vi "Saving Ascan data.vi"(8 "error in (no error)":errorcluster caption="错误输入（无错误）", 10 "Ascan Data":dbl[](array[numeric]) caption="第一行", 11 "名称或相对路径":string) -> (0 "error out":errorcluster caption="错误输出")   [LabVIEW 2015, in "Utility VIs.lvlib"]
uses:
  Utility VIs.lvlib
  <vilib>/Utility/file.llb/Write Delimited Spreadsheet (DBL).vi
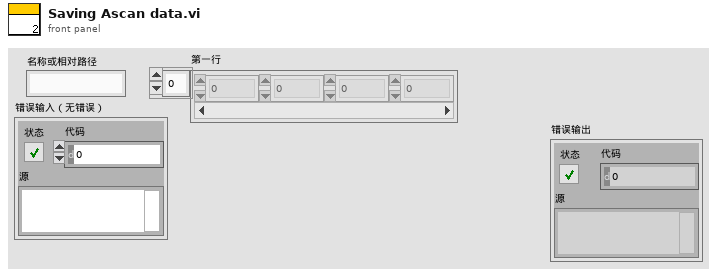
[diagram p1: front panel]
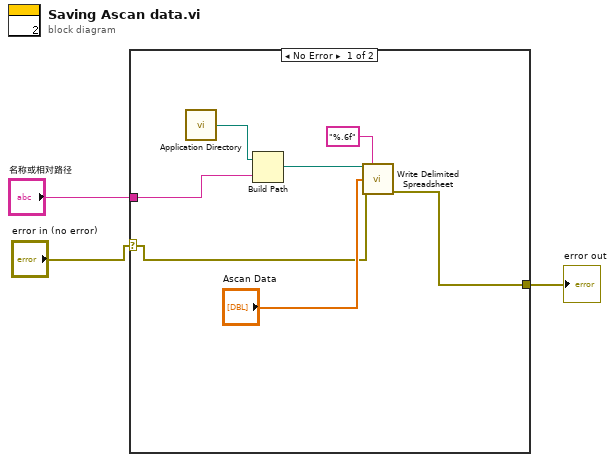
[diagram p0: block diagram]
diagram:
  n1 = case shown="No Error" "error in (no error)" {
    selector: "error in (no error)" -> [w5 w11]
    tunnel: "名称或相对路径" -> [w9 _]
    tunnel: [w7 w11] -> w2
    frame No Error {
      n2 = call <vilib>:"Application Directory.vi"() -> ("Application Directory"=w10:path)
      n3 = Build Path(base path=w10, name or relative path=w9) -> (appended path=w8:path)
      n4 = call-poly <vilib>:"Write Delimited Spreadsheet.vi"("file path (dialog if empty)"=w8, "format (%.3f)"="%.6f", "1D data"="Ascan Data", "error in (no error)"=w5) -> ("error out"=w7:errorcluster)  [unwired: 10 in, 1 out]
    }
    frame Error {
    }
  }
  "error out" <- w2
